vi "Test Tektronix.vi"() -> ()   [LabVIEW 2020, in "Tektronicks.lvclass"]
uses:
  Tektronicks.lvclass
  TypeDefs/ReadWaveform--cluster.ctl
  Libraries/Osciloscope/Osciloscope.lvlib
panel:
  out "Waveform Graph":dbl[](graph)
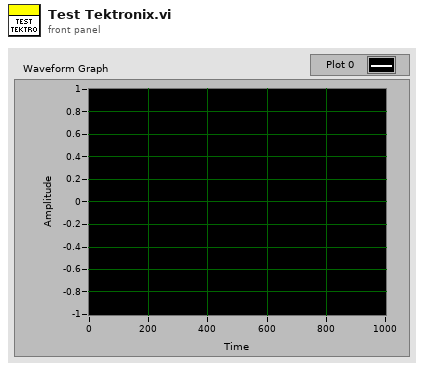
[diagram p1: front panel]
types:
  T1 = typedef "ReadWaveform--cluster.ctl" = cluster{"TEKTRONIX READ-WAVEFORM 2":cluster{"Source (0: Channel 1)":u16, "Timeout (10000 ms) 2":u32}, "EDU-X-1200A- READ-WAVEFORM":cluster{"Bind Source Channel (2: None)":i32, "Timeout (10000 ms)":u32, "Source Channel (0: Channel 1)":i32}}
  T2 = typedef "Osciloscope.lvlib/Broadcast Events--cluster.ctl" = cluster{"Module Did Init":refnum<user-event>, "Status Updated":refnum<user-event>, "Error Reported":refnum<user-event>, "Module Did Stop":refnum<user-event>, "Update Module Execution Status":refnum<user-event>, "Obtain Osciloscope Name":refnum<user-event>}
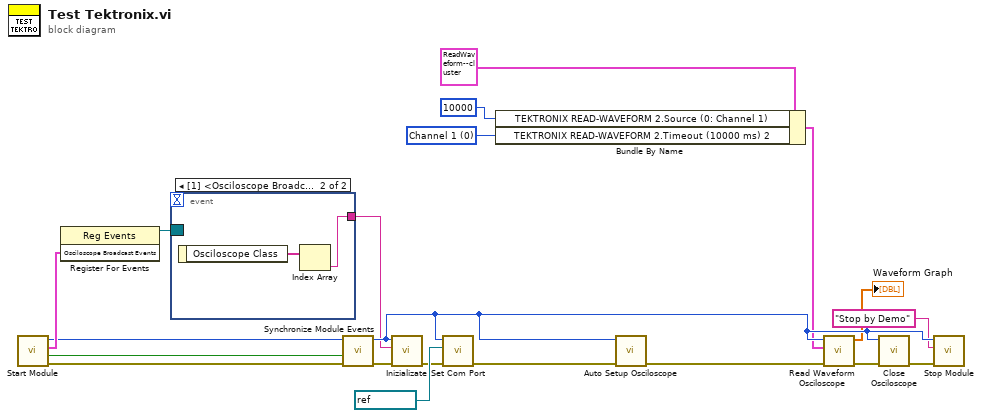
[diagram p0: block diagram]
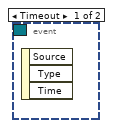
[diagram p2: hidden frame]
diagram:
  w8 = u16 0 items=["Channel 1", "Channel 2", "Channel 3", "Channel 4", "Math", "Reference A", "Reference B", "Reference C", "Reference D", "FFT"] ("Source (0: Channel 1)")
  n1 = call "Start Module.vi"() -> ("error out"=w7:errorcluster, "Wait for Event Sync?"=w18:bool, "Osciloscope Broadcast Events"=w20:T2, "Module ID"=w17:i32)  [unwired: 8 in]
  n2 = register-events(w20) -> (reference out=w19:refnum<event-registration>)  [unwired: 2 in, 1 out]
  n3 = event shown="[1] <Osciloscope Broadcast Events.Obtain Osciloscope Name>: User Event" {
    selector: w19 -> [_ _]
    dyn-events: _ -> [_ _]
    timeout: _ -> [_ _]
    tunnel: [_ w21] -> w15
    event Timeout {
      n4 = event-data() -> ()  [unwired: 1 in, 3 out]
    }
    event User Event {
      n5 = event-data() -> ("Osciloscope Class"=w22:string[])  [unwired: 1 in]
      n6 = Index Array(array=w22) -> (element=w21:string)  [unwired: 1 in]
    }
  }
  n7 = call "Synchronize Module Events.vi"("error in"=w7, "Wait for Event Sync?"=w18, "Module ID in"=w17) -> ("error out"=w6:errorcluster, "Module ID out"=w16:i32)  [unwired: 7 in]
  n8 = call "Inizializate.vi"("error in"=w6, "Osciloscope"=w15, "Module ID"=w16) -> ("error out"=w5:errorcluster)  [unwired: 8 in]
  n9 = call "Set Com Port.vi"("error in"=w5, "Com Port"=refnum<visa-resource-name> "COM1", "Module ID"=w16) -> ("error out"=w4:errorcluster)  [unwired: 8 in]
  n10 = Bundle By Name(cluster=T1 {"TEKTRONIX READ-WAVEFORM 2"={"Source (0: Channel 1)"=0, "Timeout (10000 ms) 2"=10000}, "EDU-X-1200A- READ-WAVEFORM"={"Bind Source Channel (2: None)"=2, "Timeout (10000 ms)"=10000, "Source Channel (0: Channel 1)"=0}} ("ReadWaveform"), "TEKTRONIX READ-WAVEFORM 2.Source (0: Channel 1)"=u32 10000 ("Timeout (10000 ms) 2"), "TEKTRONIX READ-WAVEFORM 2.Timeout (10000 ms) 2"=w8) -> (w11:T1)
  n11 = call "Auto Setup Osciloscope.vi"("error in"=w4, "Module ID"=w16) -> ("error out"=w3:errorcluster)  [unwired: 9 in]
  n12 = call "Read Waveform Osciloscope.vi"("error in"=w3, "ReadWaveform"=w11, "Module ID"=w16) -> ("error out"=w2:errorcluster, "Waveform Graph"=→"Waveform Graph":dbl[])  [unwired: 6 in, 1 out]
  n13 = call "Close Osciloscope.vi"("error in"=w2, "Module ID"=w16) -> ("error out"=w1:errorcluster)  [unwired: 9 in]
  n14 = call "Stop Module.vi"("error in (no error)"=w1, "Origin"="Stop by Demo", "Module ID"=w16) -> ()  [unwired: 8 in, 1 out]
